vi "Read Attributes.vi"(11 "Return DER_Measurement Msg":refnum<class "Return DER_Measurement Msg.lvclass">) -> (2 "Payload":cluster{"DER_Measurement":T1})   [LabVIEW 2018, in "EMS Generic Actor.lvlib" / "Return DER_Measurement Msg.lvclass"]
uses:
  Return DER_Measurement Msg.lvclass
  <vilib>/ORNL/CSEISMIC DDS/CSEISMIC DDS Base/Data Types/DER_Measurement.ctl
  <vilib>/ORNL/CSEISMIC DDS/CSEISMIC DDS Base/Data Types/Controls/DeviceID.ctl
  Return DER_Measurement Msg.lvclass/Return DER_Measurement Msg.ctl
  <vilib>/ORNL/CSEISMIC DDS/CSEISMIC DDS Base/CSEISMIC DDS.lvclass
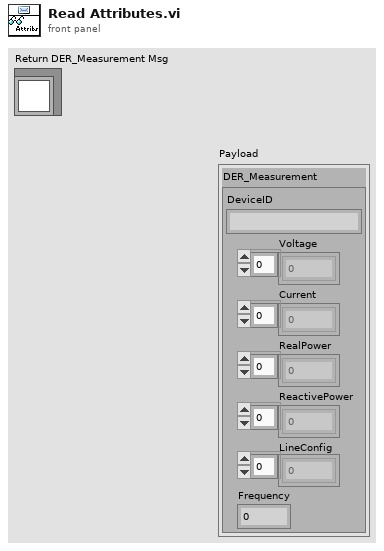
[diagram p1: front panel]
types:
  T1 = typedef "CSEISMIC DDS.lvlib/CSEISMIC DDS.lvclass/DER_Measurement.ctl" = cluster{"DeviceID":T2, "Voltage":dbl[], "Current":dbl[], "RealPower":dbl[], "ReactivePower":dbl[], "LineConfig":u8[], "Frequency":dbl}
  T2 = typedef "CSEISMIC DDS.lvlib/CSEISMIC DDS.lvclass/DeviceID.ctl" = string
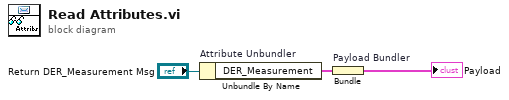
[diagram p0: block diagram]
diagram:
  n1 = Unbundle By Name "Attribute Unbundler"("Return DER_Measurement Msg") -> ("DER_Measurement"=w1:T1)
  n2 = Bundle "Payload Bundler"("DER_Measurement"=w1) -> (→"Payload":cluster{"DER_Measurement":T1})  [unwired: 1 in]
